vi "PH_BL-Master.set standard GUI element tip strip.vi"(3 "Instance Name":string="ns_Nearfield_Ring_Exit_Cam", 4 "Element State":T1=enum."No Info") -> (17 "Tip Strip":string)   [LabVIEW 2014, in "PH_BL-Master.lvlib"]
doc: "Within this VI the tip strip of an object is set; \n\n@ Default: \"<Instance Name> not linked yet\n\n@ No Info: \"<Instance Name> \n no info\" \n\n@ IN: \"<Instance Name> is running \n at <System ID> on <Node>.\""
uses:
  PH_BL-Master.lvlib
  PH_BL-Master.Shutter State.ctl
  CSCore/CSSystem/CSSystemLib/CSSystemLib.lvlib
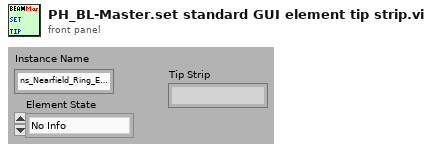
[diagram p1: front panel]
types:
  T1 = typedef "PH_BL-Master.lvlib/PH_BL-Master.Shutter State.ctl" = enum16{"No Link", "No Info", "In", "Out", "in between"}
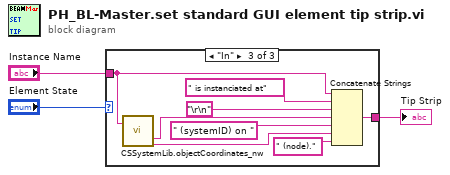
[diagram p0: block diagram]
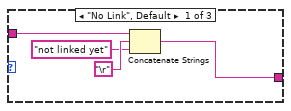
[diagram p2: hidden frame]
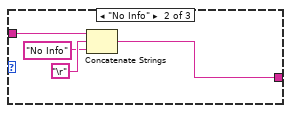
[diagram p3: hidden frame]
diagram:
  n1 = case shown="\"In\"" "Element State" {
    tunnel: "Instance Name" -> [w6 w9 w15]
    tunnel: [w7 w8 w12] -> w2
    frame "No Link", Default {
      n2 = Concatenate Strings(w6, "\r", "not linked yet") -> (w7:string)
    }
    frame "No Info" {
      n3 = Concatenate Strings(w9, "\r", "No Info") -> (w8:string)
    }
    frame "In" {
      n4 = call "CSSystemLib.objectCoordinates_nw.vi"("name"=w15) -> ("systemID"=w14:string, "node"=w13:string)  [unwired: 15 in, 2 out]
      n5 = Concatenate Strings(w15, " is instanciated at", "\r\n", w14, " (systemID) on ", w13, " (node).") -> (w12:string)
    }
  }
  "Tip Strip" <- w2
